vi "make_synth_array (SubVI).vi"(1 "Synth settings:":T1={"start volt (V)"=1.0, "stop volt (V) "=1.0, "# V Steps"=1, "start freq (Hz)"=2000.0, "stop freq (Hz) "=2000.0, "# F steps"=1, "dc offset?"=FALSE, "start DC (V)"=0.5, "stop DC (V)"=0.5, "# DC steps "=1, "Set synth\n(HP33120A)?"=FALSE, "Use arbitrary\nwaveform?"=FALSE, "Arb waveform name:"=""}) -> (0 "Tot Synth Arr":dbl[][](array[numeric]))   [LabVIEW 2018]
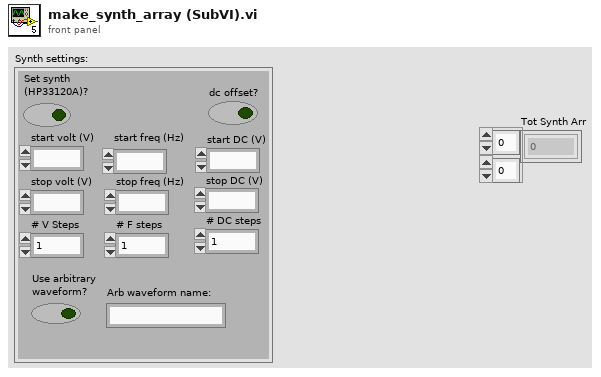
[diagram p1: front panel]
types:
  T1 = cluster{"start volt (V)":ext, "stop volt (V) ":ext, "# V Steps":i32, "start freq (Hz)":ext, "stop freq (Hz) ":ext, "# F steps":i32, "dc offset?":bool, "start DC (V)":ext, "stop DC (V)":ext, "# DC steps ":i32, "Set synth\n(HP33120A)?":bool, "Use arbitrary\nwaveform?":bool, "Arb waveform name:":string}
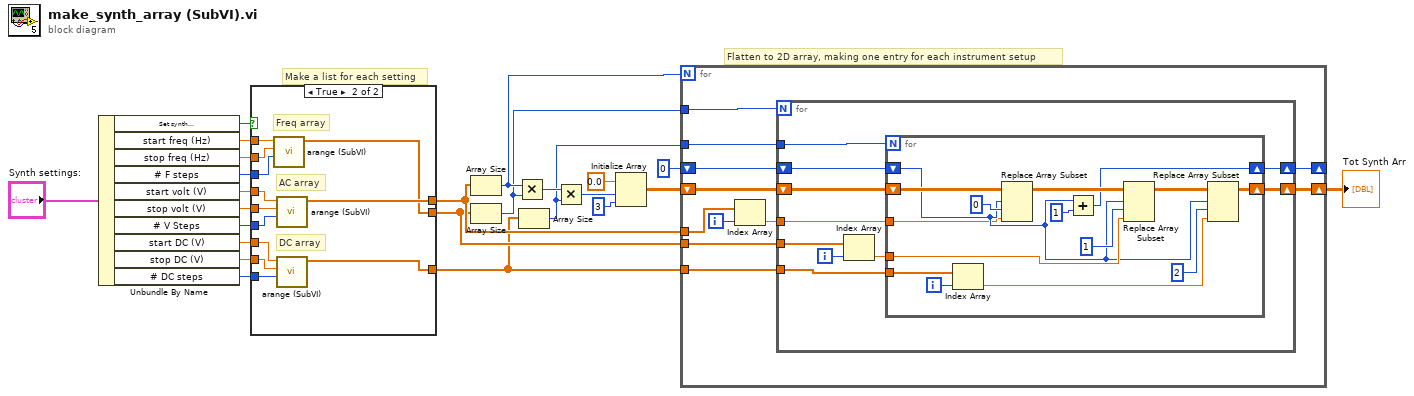
[diagram p0: block diagram]
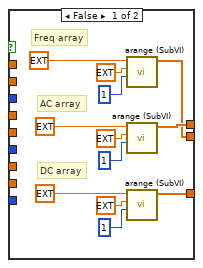
[diagram p2: hidden frame]
diagram:
  # "Make a list for each setting"
  # "Flatten to 2D array, making one entry for each instrument setup"
  n1 = Unbundle By Name("Synth settings:") -> ("Set synth\n(HP33120A)?"=w7:bool, "start freq (Hz)"=w6:ext, "stop freq (Hz)"=w5:ext, "# F steps"=w4:i32, "start volt (V)"=w3:ext, "stop volt (V)"=w2:ext, "# V Steps"=w1:i32, "start DC (V)"=w24:ext, "stop DC (V)"=w23:ext, "# DC steps"=w22:i32)
  n2 = case shown="True" w7 {
    tunnel: w3 -> [_ w48]
    tunnel: w2 -> [_ w47]
    tunnel: w1 -> [_ w46]
    tunnel: w6 -> [_ w45]
    tunnel: w5 -> [_ w44]
    tunnel: w4 -> [_ w43]
    tunnel: w24 -> [_ w42]
    tunnel: w23 -> [_ w41]
    tunnel: w22 -> [_ w40]
    tunnel: [w27 w39] -> w14
    tunnel: [w26 w38] -> w13
    tunnel: [w25 w37] -> w12
    frame False {
      # "DC array"
      # "Freq array"
      # "AC array"
      n3 = call "arange (SubVI).vi"("# Steps"=1, "stop"=ext -1.0, "start"=ext -1.0) -> ("Array"=w26:ext[])  [unwired: 8 in]
      n4 = call "arange (SubVI).vi"("# Steps"=1, "stop"=ext -1.0, "start"=ext -1.0) -> ("Array"=w27:ext[])  [unwired: 8 in]
      n5 = call "arange (SubVI).vi"("# Steps"=1, "stop"=ext -1.0, "start"=ext -1.0) -> ("Array"=w25:ext[])  [unwired: 8 in]
    }
    frame True {
      # "DC array"
      # "Freq array"
      # "AC array"
      n6 = call "arange (SubVI).vi"("# Steps"=w43, "stop"=w44, "start"=w45) -> ("Array"=w38:ext[])  [unwired: 8 in]
      n7 = call "arange (SubVI).vi"("# Steps"=w46, "stop"=w47, "start"=w48) -> ("Array"=w39:ext[])  [unwired: 8 in]
      n8 = call "arange (SubVI).vi"("# Steps"=w40, "stop"=w41, "start"=w42) -> ("Array"=w37:ext[])  [unwired: 8 in]
    }
  }
  n9 = Array Size(array=w14) -> (size(s)=w11:i32)
  n10 = Array Size(array=w13) -> (size(s)=w10:i32)
  n11 = Multiply(x=w11, y=w10) -> (x*y=w20:i32)
  n12 = Array Size(array=w12) -> (size(s)=w9:i32)
  n13 = Multiply(x=w20, y=w9) -> (x*y=w19:i32)
  n14 = Initialize Array(0.0 ("element"), w19, 3 ("dimension size")) -> (w17:dbl[][])
  n15 = for {
    N: w11 -> [_]
    shift-right: [w49] -> _
    shift-left: 0 ("disabled index (row)") -> [w50]
    shift-right: [w58] -> w15
    shift-left: w17 -> [w59]
    tunnel: w14 -> [w57]
    tunnel: w13 -> [w54]
    tunnel: w12 -> [w53]
    tunnel: w10 -> [w52]
    tunnel: w9 -> [w51]
    i -> [w55]
    n16 = Index Array(array=w57, index=w55) -> (element=w56:ext)
    n17 = for {
      N: w52 -> [_]
      tunnel: w56 -> [w67]
      tunnel: w54 -> [w66]
      tunnel: w53 -> [w63]
      tunnel: w51 -> [w62]
      shift-right: [w68] -> w58
      shift-left: w59 -> [w69]
      shift-right: [w60] -> w49
      shift-left: w50 -> [w61]
      i -> [w65]
      n18 = Index Array(array=w66, index=w65) -> (element=w64:ext)
      n19 = for {
        N: w62 -> [_]
        tunnel: w67 -> [w70]
        tunnel: w64 -> [w77]
        tunnel: w63 -> [w75]
        shift-right: [w80] -> w68
        shift-left: w69 -> [w84]
        shift-right: [w72] -> w60
        shift-left: w61 -> [w71]
        i -> [w76]
        n20 = Index Array(array=w75, index=w76) -> (element=w74:ext)
        n21 = Replace Array Subset(array=w84, new element=w70, index (row)=w71, index (col)=0 ("disabled index (col)")) -> (w82:dbl[][])
        n22 = Add(x=w71, y=1) -> (x+y=w72:i32)
        n23 = Replace Array Subset(array=w82, new element=w77, index (row)=w71, index (col)=1 ("disabled index (col)")) -> (w81:dbl[][])
        n24 = Replace Array Subset(array=w81, new element=w74, index (row)=w71, index (col)=2 ("disabled index (col)")) -> (w80:dbl[][])
      }
    }
  }
  "Tot Synth Arr" <- w15
